vi "Diff_Drive_Pose_Estimation_Tracking.vi"() -> ()   [LabVIEW 2019]
uses:
  <vilib>/Rock Robotics/WPI/Joystick/WPI_JoystickArcadeMapping.vi
  Sim_Diff_Drive_Globals.vi
panel:
  in  "Force Multiplier":dbl
  in  "Angular Throttle":dbl(slide) scale=-1.0..1.0
  in  "Linear Throttle":dbl(slide) scale=-1.0..1.0
  in  "stop":bool
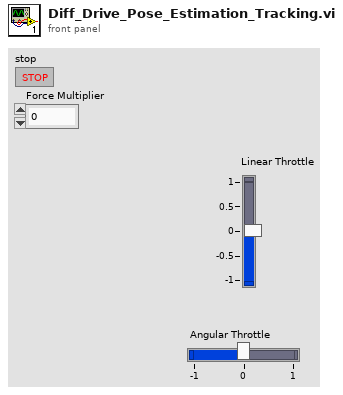
[diagram p1: front panel]
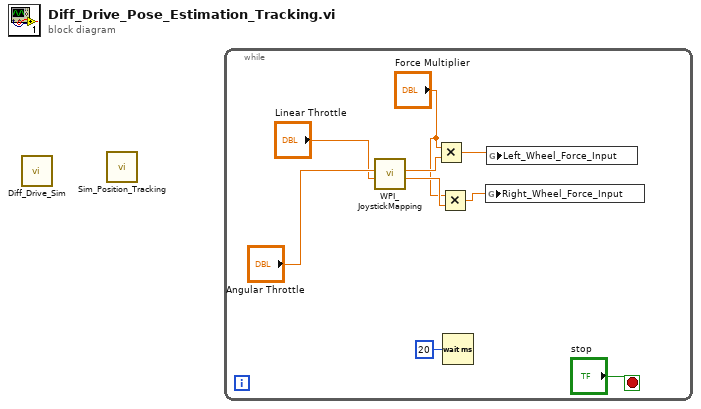
[diagram p0: block diagram]
diagram:
  n1 = call "Diff_Drive_Sim.vi"() -> ()  [unwired: 12 in]
  n2 = call "Sim_Position_Tracking.vi"() -> ()  [unwired: 12 in]
  n3 = while {
    stop <- "stop" stop-if-true
    n4 = call-poly <vilib>:"WPI_JoystickMapping.vi"("Y axis value"="Linear Throttle", "X axis value"="Angular Throttle") -> ("Right Motor Value"=w2:dbl, "Left Motor Value"=w4:dbl)  [unwired: 8 in]
    n5 = Multiply(x="Force Multiplier", y=w4) -> (x*y=w5:dbl)
    n6 = Multiply(x="Force Multiplier", y=w2) -> (x*y=w3:dbl)
    n7 = Wait (ms)(milliseconds to wait=u32 20) -> ()  [unwired: 1 out]
    n8 = global write "Sim_Diff_Drive_Globals.vi" "Right_Wheel_Force_Input"(w3) -> ()
    n9 = global write "Sim_Diff_Drive_Globals.vi" "Left_Wheel_Force_Input"(w5) -> ()
  }
